vi "GCP_Foot_L.vi"(10 "threshold":T1={"High 검출값"=400.0, "Low 기준값"=-400.0, "MID 중간값"=-200.0}, 11 "Foot Angular velocity":sgl) -> (0 "L_Ctrl_Start":bool, 1 "L_Period":u32, 2 "L_GCP":dbl, 3 "L_num":u32)   [LabVIEW 2019]
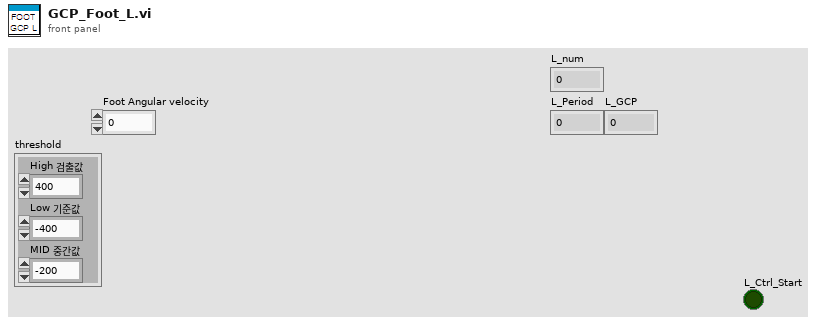
[diagram p1: front panel]
types:
  T1 = cluster{"High 검출값":sgl, "Low 기준값":sgl, "MID 중간값":sgl}
  T2 = enum16{"Init", "MS", "SE", "HS", "FF", "TO", "SS"}
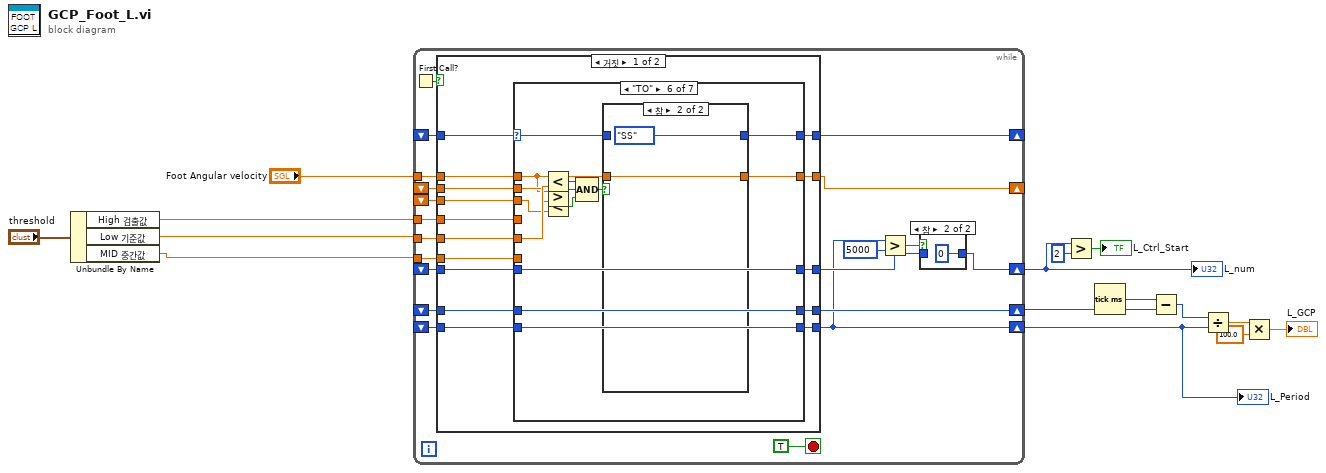
[diagram p0: block diagram]
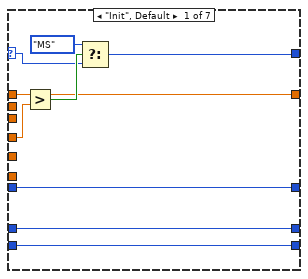
[diagram p3: hidden frame]
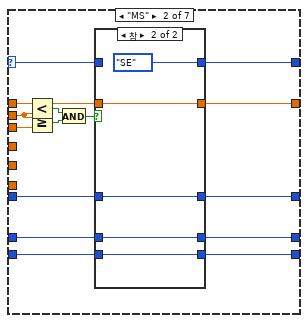
[diagram p4: hidden frame]
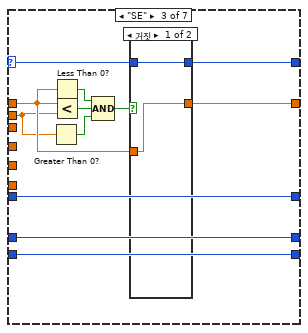
[diagram p6: hidden frame]
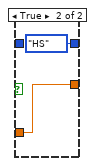
[diagram p7: hidden frame]
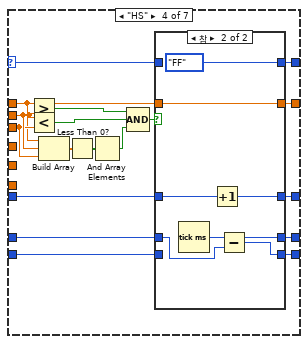
[diagram p8: hidden frame]
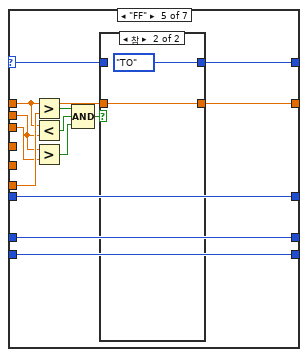
[diagram p10: hidden frame]
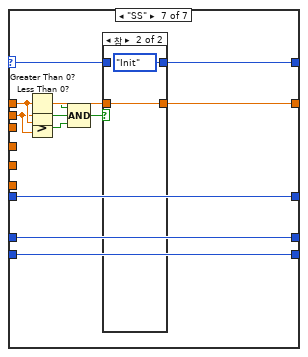
[diagram p13: hidden frame]
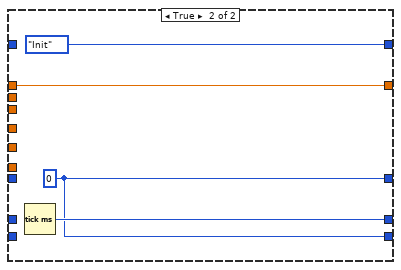
[diagram p15: hidden frame]
diagram:
  n1 = Unbundle By Name("threshold") -> ("High 검출값"=w3:sgl, "Low 기준값"=w2:sgl, "MID 중간값"=w1:sgl)
  n2 = while {
    tunnel: w3 -> [w31]
    tunnel: w2 -> [w23]
    shift-right: [w33] -> _
    shift-left: _ -> [w32]
    shift-right: [w24] -> _
    shift-left: _ -> [w30]
    shift-left: _ -> [w29]
    shift-right: [w17] -> w5
    shift-left: _ -> [w28]
    shift-right: [w27] -> w13
    shift-left: _ -> [w26]
    shift-right: [w16] -> w11
    shift-left: _ -> [w25]
    tunnel: "Foot Angular velocity" -> [w22]
    tunnel: w1 -> [w21]
    stop <- TRUE stop-if-true
    n3 = First Call?() -> (First Call?: T/F=w34:bool)
    n4 = case shown="거짓" w34 {
      tunnel: [w49 T2."Init"] -> w33
      tunnel: w32 -> [w52 _]
      tunnel: w22 -> [w51 w185]
      tunnel: w31 -> [w50 _]
      tunnel: w30 -> [w48 _]
      tunnel: w29 -> [w47 _]
      tunnel: [w46 w186] -> w18
      tunnel: w28 -> [w45 _]
      tunnel: [w44 w187] -> w27
      tunnel: w26 -> [w43 _]
      tunnel: [w42 w186] -> w16
      tunnel: w25 -> [w41 _]
      tunnel: [w40 w185] -> w24
      tunnel: w23 -> [w39 _]
      tunnel: w21 -> [w38 _]
      frame False {
        n5 = case shown="\"TO\"" w52 {
          selector: w52 -> [w59 w68 w98 w113 w146 w156 w178]
          tunnel: w51 -> [w54 w63 w92 w112 w142 w152 w180]
          tunnel: w50 -> [w61 _ _ _ _ _ _]
          tunnel: [w58 w71 w97 w114 w145 w157 w179] -> w49
          tunnel: w48 -> [_ w76 w91 w118 w141 w163 w177]
          tunnel: w47 -> [_ w75 _ w117 w140 w162 _]
          tunnel: [w57 w70 w96 w103 w135 w155 w172] -> w46
          tunnel: w45 -> [w57 w69 w96 w104 w135 w155 w172]
          tunnel: [w56 w67 w95 w106 w134 w154 w171] -> w44
          tunnel: w43 -> [w56 w66 w95 w108 w134 w154 w171]
          tunnel: [w55 w65 w94 w105 w133 w153 w170] -> w42
          tunnel: w41 -> [w55 w64 w94 w107 w133 w153 w170]
          tunnel: [w54 w62 w93 w111 w144 w151 w169] -> w40
          tunnel: w39 -> [_ _ _ _ _ w164 _]
          tunnel: w38 -> [_ _ _ _ w143 _ _]
          frame "Init", Default {
            n6 = Greater?(x=w54, y=w61) -> (0:w60:bool)
            n7 = Select(t=T2."MS", s=w60, f=w59) -> (s? t:f=w58:T2)
          }
          frame "MS" {
            n8 = Less?(x=w63, y=w76) -> (x < y?=w74:bool)
            n9 = Greater Or Equal?(x=w76, y=w75) -> (x >= y?=w73:bool)
            n10 = And(x=w74, y=w73) -> (x .and. y?=w72:bool)
            n11 = case shown="참" w72 {
              tunnel: [w80 T2."SE"] -> w71
              tunnel: [w81 w84] -> w70
              tunnel: w69 -> [w81 w84]
              tunnel: w68 -> [w80 _]
              tunnel: [w79 w83] -> w67
              tunnel: w66 -> [w79 w83]
              tunnel: [w78 w82] -> w65
              tunnel: w64 -> [w78 w82]
              tunnel: [w77 w86] -> w62
              tunnel: w63 -> [w77 w86]
              frame False {
              }
              frame True {
              }
            }
          }
          frame "SE" {
            n12 = Greater Than 0?(x=w91) -> (x > 0?=w88:bool)
            n13 = Less Than 0?(x=w92) -> (x < 0?=w90:bool)
            n14 = Less?(x=w92, y=w91) -> (x < y?=w89:bool)
            n15 = Compound Arithmetic op=AND ("복합 연산")(w90, w89, w88) -> (w87:bool)
            n16 = case shown="거짓" w87 {
              tunnel: w98 -> [w100 _]
              tunnel: [w100 T2."HS"] -> w97
              tunnel: w92 -> [w99 w102]
              tunnel: [w99 w102] -> w93
              frame False {
              }
              frame True {
              }
            }
          }
          frame "HS" {
            n17 = Greater?(x=w112, y=w118) -> (0:w120:bool)
            n18 = Less?(x=w118, y=w117) -> (x < y?=w119:bool)
            n19 = Build Array(w112, w118, w117) -> (w116:sgl[])
            n20 = Less Than 0?(x=w116) -> (x < 0?=w115:bool[])
            n21 = And Array Elements(Boolean array=w115) -> (logical AND=w109:bool)
            n22 = Compound Arithmetic op=AND ("복합 연산")(w120, w119, w109) -> (w110:bool)
            n23 = case shown="참" w110 {
              tunnel: [w125 T2."FF"] -> w114
              tunnel: w113 -> [w125 _]
              tunnel: w112 -> [w124 w132]
              tunnel: [w124 w132] -> w111
              tunnel: w108 -> [w123 w128]
              tunnel: w107 -> [w122 _]
              tunnel: [w123 w130] -> w106
              tunnel: [w122 w129] -> w105
              tunnel: w104 -> [w121 w127]
              tunnel: [w121 w126] -> w103
              frame False {
              }
              frame True {
                n24 = Tick Count (ms)() -> (millisecond timer value=w130:u32)
                n25 = Increment(x=w127) -> (x+1=w126:u32)
                n26 = Subtract(x=w130, y=w128) -> (x-y=w129:u32)
              }
            }
          }
          frame "FF" {
            n27 = Greater?(x=w142, y=w143) -> (0:w139:bool)
            n28 = Less?(x=w142, y=w141) -> (x < y?=w138:bool)
            n29 = Greater?(x=w141, y=w140) -> (0:w137:bool)
            n30 = Compound Arithmetic op=AND ("복합 연산")(w139, w138, w137) -> (w136:bool)
            n31 = case shown="참" w136 {
              tunnel: w146 -> [w147 _]
              tunnel: [w147 T2."TO"] -> w145
              tunnel: [w148 w149] -> w144
              tunnel: w142 -> [w148 w149]
              frame False {
              }
              frame True {
              }
            }
          }
          frame "TO" {
            n32 = Less?(x=w152, y=w164) -> (x < y?=w161:bool)
            n33 = Greater?(x=w152, y=w163) -> (0:w160:bool)
            n34 = Less?(x=w163, y=w162) -> (x < y?=w159:bool)
            n35 = Compound Arithmetic op=AND ("복합 연산")(w161, w160, w159) -> (w158:bool)
            n36 = case shown="참" w158 {
              tunnel: [w166 T2."SS"] -> w157
              tunnel: w156 -> [w166 _]
              tunnel: w152 -> [w165 w168]
              tunnel: [w165 w168] -> w151
              frame False {
              }
              frame True {
              }
            }
          }
          frame "SS" {
            n37 = Greater Than 0?(x=w180) -> (x > 0?=w176:bool)
            n38 = Less Than 0?(x=w177) -> (x < 0?=w175:bool)
            n39 = Greater?(x=w180, y=w177) -> (0:w174:bool)
            n40 = Compound Arithmetic op=AND ("복합 연산")(w176, w175, w174) -> (w173:bool)
            n41 = case shown="참" w173 {
              tunnel: [w182 T2."Init"] -> w179
              tunnel: w178 -> [w182 _]
              tunnel: w180 -> [w181 w184]
              tunnel: [w181 w184] -> w169
              frame False {
              }
              frame True {
              }
            }
          }
        }
      }
      frame True {
        w186 = u32 0
        n42 = Tick Count (ms)() -> (millisecond timer value=w187:u32)
      }
    }
    n43 = Greater?(x=w16, y=u32 5000) -> (0:w20:bool)
    n44 = case shown="참" w20 {
      tunnel: [w36 u32 0] -> w17
      tunnel: w18 -> [w36 _]
      frame False {
      }
      frame True {
      }
    }
  }
  "L_num" <- w5
  "L_Period" <- w11
  n45 = Greater?(x=w5, y=u32 2) -> (0:→"L_Ctrl_Start":bool)
  n46 = Tick Count (ms)() -> (millisecond timer value=w14:u32)
  n47 = Subtract(x=w14, y=w13) -> (x-y=w12:u32)
  n48 = Divide(x=w12, y=w11) -> (x/y=w10:dbl)
  n49 = Multiply(x=w10, y=100.0) -> (x*y=→"L_GCP":dbl)
